vi "CenterPoint.vi"(8 "error in (no error)":errorcluster, 11 "IDrawable in":refnum<class "IDrawable.lvclass">) -> (0 "error out":errorcluster, 2 "CenterPoint":refnum<class "Point.lvclass">, 3 "IDrawable out":refnum<class "IDrawable.lvclass">)   [LabVIEW 2021, in "Picture2D.lvlib" / "IDrawable.lvclass"]
uses:
  IDrawable.lvclass
  Point/Point.lvclass
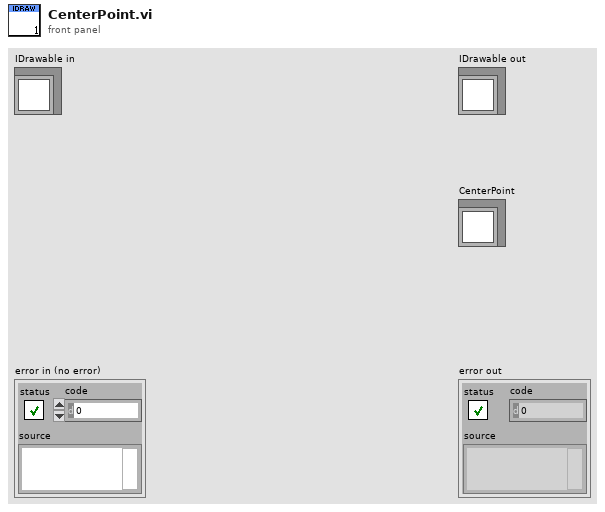
[diagram p1: front panel]
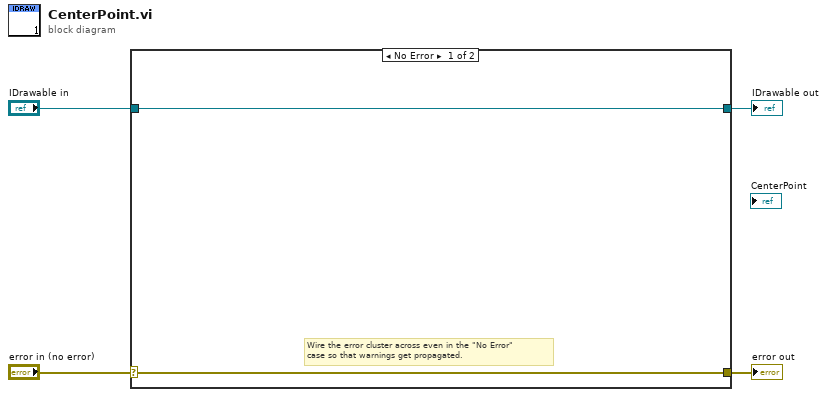
[diagram p0: block diagram]
diagram:
  n1 = case shown="No Error" "error in (no error)" {
    selector: "error in (no error)" -> [w5 w8]
    tunnel: [w5 w8] -> w3
    tunnel: [w6 w7] -> w1
    tunnel: "IDrawable in" -> [w6 w7]
    frame No Error {
      # "Wire the error cluster across even in the \"No Error\"\ncase so that warnings get propagated."
    }
    frame Error {
    }
  }
  "error out" <- w3
  "IDrawable out" <- w1
